vi "Test Animal Cannot Sleep when Hungry.vi"(8 "error in (no error)":errorcluster, 11 "Animal Test in":refnum<class "Animal Test.lvclass">) -> (0 "error out":errorcluster, 3 "Animal Test out":refnum<class "Animal Test.lvclass">)   [LabVIEW 2020, in "Animal Test.lvclass"]
doc: "Test Animal cannot sleep when hungry."
uses:
  Animal Test.lvclass
  C:/Program Files (x86)/National Instruments/LabVIEW 2020/vi.lib/Astemes/LUnit/Test Case.lvclass
  Animal Test.lvclass/Animal Test.ctl
  <vilib>/Astemes/LUnit/Test Case.lvclass/Test Case.ctl
  32eb666c-557e-449b-99dc-a8e40f1cda57.vi
  <vilib>/Astemes/LUnit/Append Fail Result.vi
  <vilib>/Astemes/LUnit/Append Pass Result.vi
  <vilib>/Astemes/LUnit/Compare Variants.vi
  <vilib>/Astemes/LUnit/Describe Comparison.vi
  <vilib>/Astemes/LUnit/Run In UI.vi
  <vilib>/Utility/error.llb/Clear Errors.vi
  <vilib>/Astemes/LUnit/Describe Variant.vi
  Animal Classes/Animal/Animal.lvclass
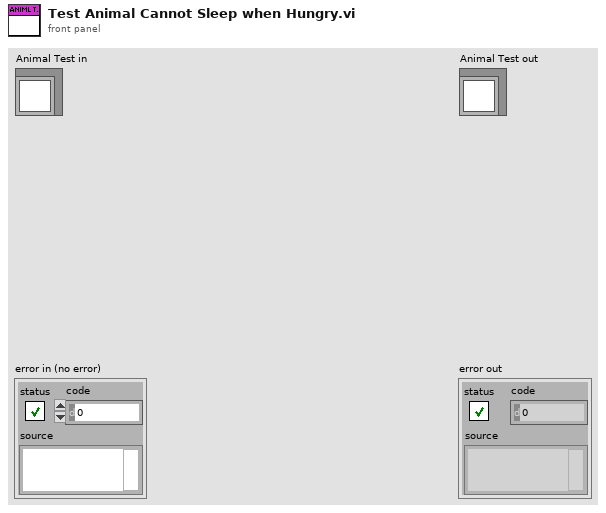
[diagram p1: front panel]
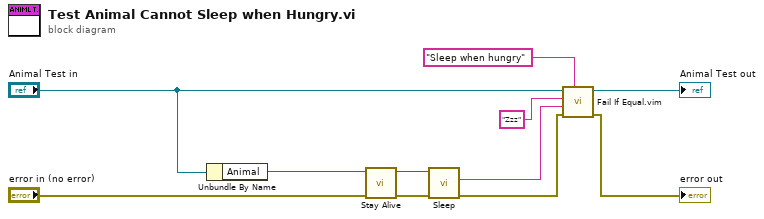
[diagram p0: block diagram]
diagram:
  n1 = Unbundle By Name("Animal Test in") -> ("Animal"=w9:refnum<class "Animal.lvclass">)
  n2 = call-dynamic "Stay Alive.vi"("error in (no error)"="error in (no error)", "Animal in"=w9) -> ("error out"=w10:errorcluster, "Animal out"=w11:refnum<class "Animal.lvclass">)  [unwired: 8 in]
  n3 = call-dynamic "Sleep.vi"("error in (no error)"=w10, "Animal in"=w11) -> ("error out"=w3:errorcluster, "Result"=w5:string)  [unwired: 7 in, 1 out]
  n4 = call "Fail If Equal.vim"("Description"="Sleep when hungry", "error in (no error)"=w3, "Actual"=w5, "Unexpected"="Zzz" ("Result"), "LUnit Test Case In"="Animal Test in") -> ("error out"=→"error out":errorcluster, "LUnit Test Case Out"=→"Animal Test out":refnum<class "Animal Test.lvclass">)  [unwired: 5 in]
